vi "Shut Down Device.vi"(8 "error in (no error)":errorcluster, 11 "Orca-Flash 4.0 in":refnum<class "Orca-Flash 4.0 V2.lvclass">) -> (0 "error out":errorcluster, 3 "Orca-Flash 4.0 out":refnum<class "Orca-Flash 4.0 V2.lvclass">)   [LabVIEW 2018, in "Orca-Flash 4.0 V2.lvlib" / "Orca-Flash 4.0 V2.lvclass"]
uses:
  Orca-Flash 4.0 V2.lvclass
  Orca-Flash 4.0 V2.lvclass/Orca-Flash 4.0 V2.ctl
  Resources/GLOBAL/GLOBAL Time-critical.vi
  Camera/Camera.lvclass
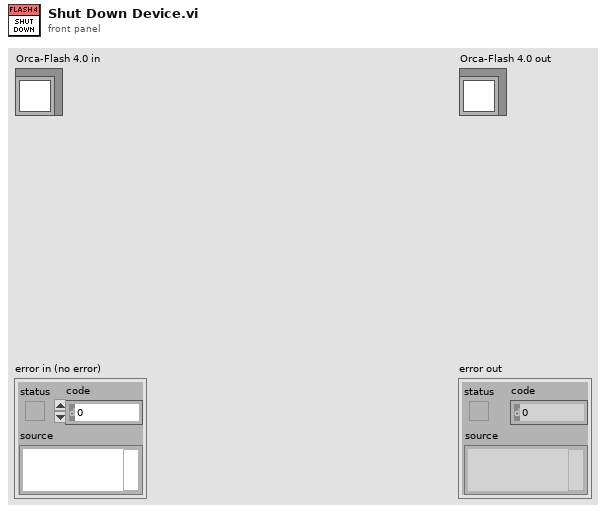
[diagram p1: front panel]
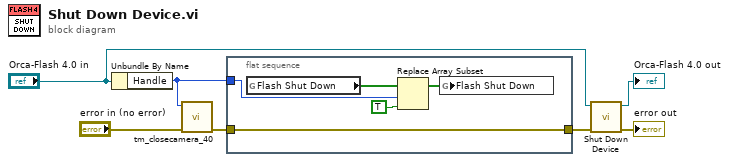
[diagram p0: block diagram]
diagram:
  n1 = Unbundle By Name("Orca-Flash 4.0 in") -> ("Handle"=w1:u32)
  n2 = call <userlib>:"tm_closecamera_40.vi"("error in (no error)"="error in (no error)", "Handle in"=w1) -> ("error out"=w2:errorcluster)  [unwired: 9 in]
  n3 = flat-sequence {
    tunnel: w2 -> [w12]
    tunnel: [w12] -> w4
    tunnel: w1 -> [w9]
    frame #0 {
      n4 = global read "GLOBAL Time-critical.vi" "Flash Shut Down"() -> (w11:bool[])
      n5 = Replace Array Subset(array=w11, new element=TRUE ("new element/subarray"), index=w9) -> (w10:bool[])
      n6 = global write "GLOBAL Time-critical.vi" "Flash Shut Down"(w10) -> ()
    }
  }
  n7 = call-parent "Shut Down Device.vi"("error in (no error)"=w4, "Device in"="Orca-Flash 4.0 in") -> ("error out"=→"error out":errorcluster, "Device out"=→"Orca-Flash 4.0 out":refnum<class "Orca-Flash 4.0 V2.lvclass">)  [unwired: 8 in]
